vi "potentially create appended path.vi"(7 "base path":path, 8 "error in (no error)":errorcluster, 9 "File name":string, 10 "Boolean":bool, 11 "DAQOrcaFlash in":refnum<class "DAQOrcaFlash.lvclass">) -> (0 "error out":errorcluster, 2 "file path":path, 3 "DAQOrcaFlash out":refnum<class "DAQOrcaFlash.lvclass">)   [LabVIEW 2012, in "DAQOrcaFlash.lvclass"]
uses:
  DAQOrcaFlash.lvclass
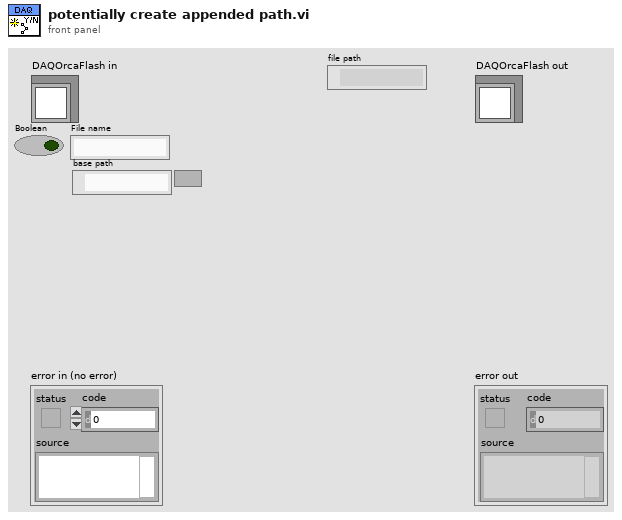
[diagram p1: front panel]
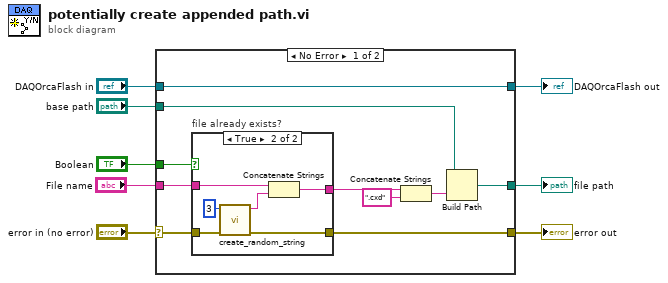
[diagram p0: block diagram]
diagram:
  n1 = case shown="No Error" "error in (no error)" {
    selector: "error in (no error)" -> [w16 w28]
    tunnel: [w17 w28] -> w7
    tunnel: [w18 w27] -> w5
    tunnel: "DAQOrcaFlash in" -> [w18 w27]
    tunnel: "Boolean" -> [w15 _]
    tunnel: "File name" -> [w14 _]
    tunnel: "base path" -> [w11 _]
    tunnel: [w9 _] -> w1
    frame No Error {
      n2 = case "file already exists?" shown="True" w15 {
        tunnel: [w20 w25] -> w17
        tunnel: w16 -> [w20 w26]
        tunnel: w14 -> [w19 w22]
        tunnel: [w19 w21] -> w13
        frame False {
        }
        frame True {
          n3 = call "create_random_string.vi"("error in (no error)"=w26, "length"=3) -> ("error out"=w25:errorcluster, "random string"=w23:string)  [unwired: 8 in]
          n4 = Concatenate Strings(w22, w23) -> (w21:string)
        }
      }
      n5 = Concatenate Strings(w13, ".cxd" ("string")) -> (w10:string)
      n6 = Build Path(base path=w11, name or relative path=w10) -> (appended path=w9:path)
    }
    frame Error {
    }
  }
  "error out" <- w7
  "DAQOrcaFlash out" <- w5
  "file path" <- w1
